vi "EnergyLevelsStatic.vi"(10 "Up/Down Control":bool=TRUE) -> (1 "Energy Level":picture)   [LabVIEW 2023]
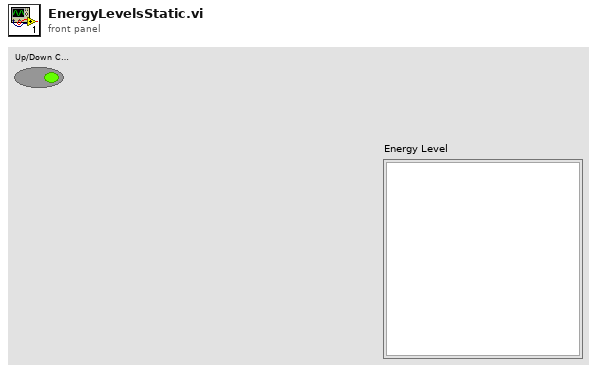
[diagram p1: front panel]
types:
  T1 = cluster{cluster{i32, i32}, cluster{i32, i32}, cluster{i32, i32}, cluster{i32, i32}}
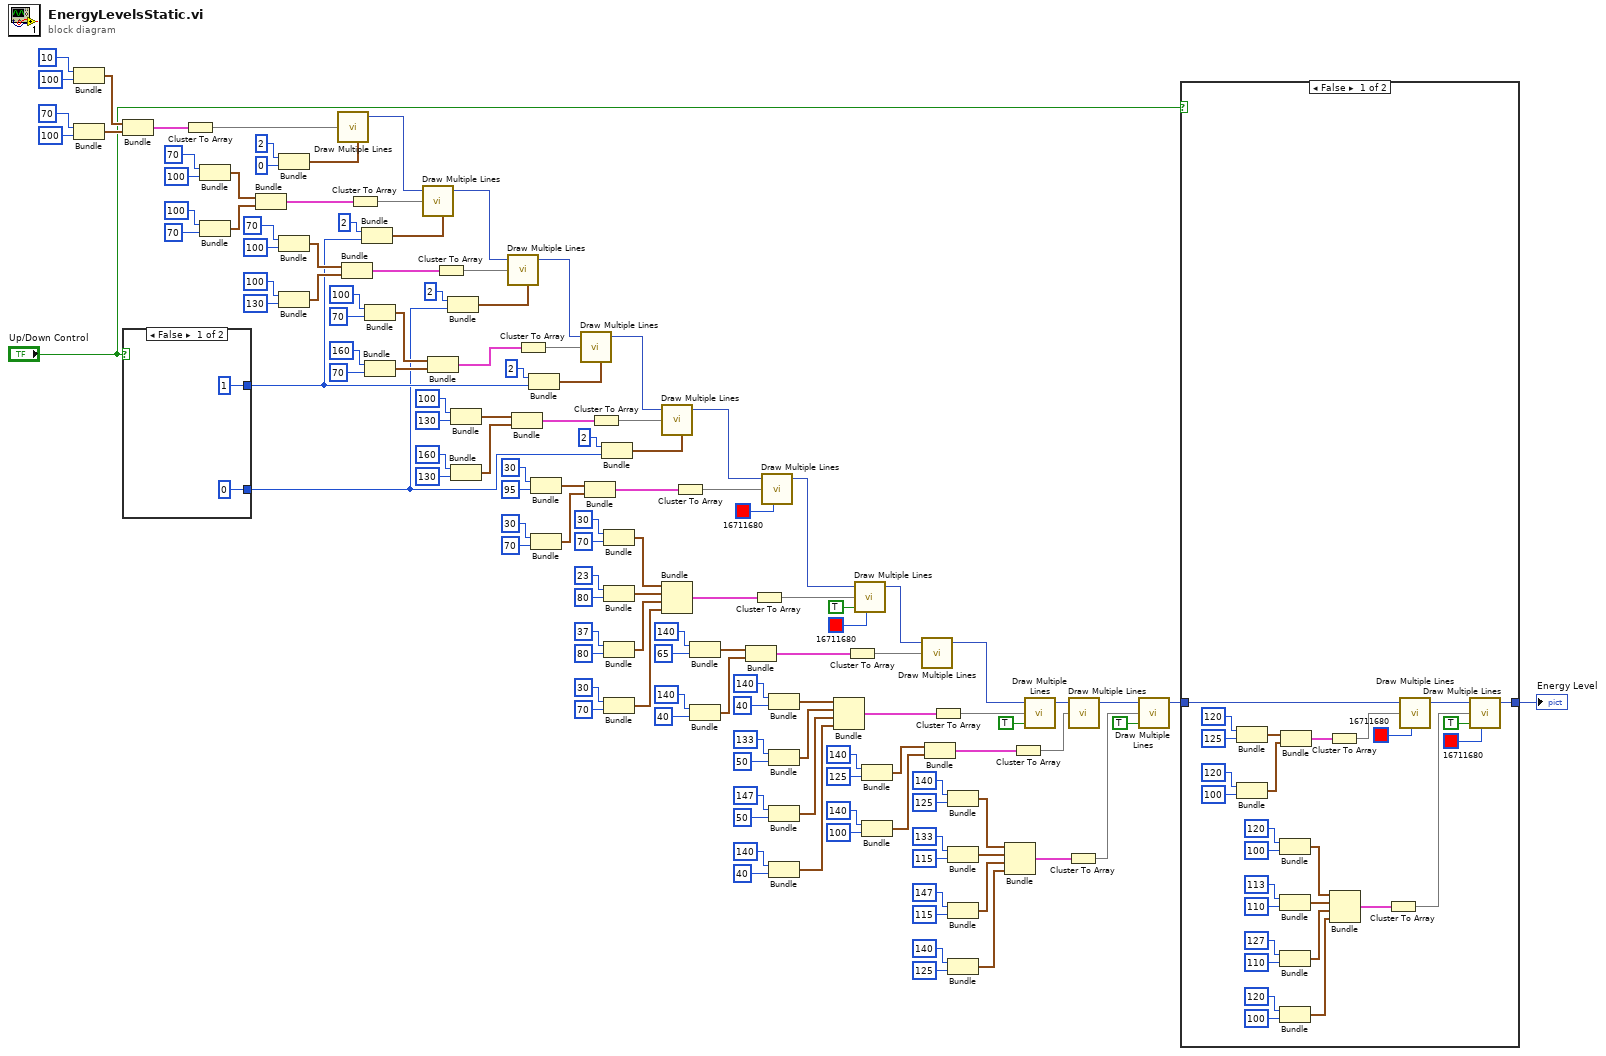
[diagram p0: block diagram]
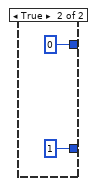
[diagram p2: hidden frame]
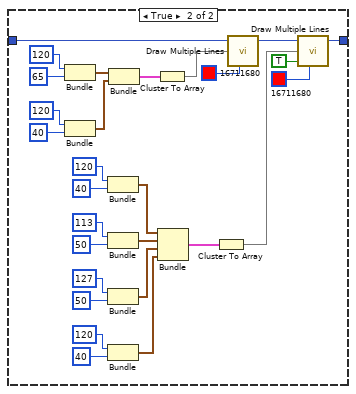
[diagram p3: hidden frame]
diagram:
  n1 = Bundle(10, 100) -> (w137:cluster{i32, i32})  [unwired: 1 in]
  n2 = Bundle(70, 100) -> (w136:cluster{i32, i32})  [unwired: 1 in]
  n3 = Bundle(w137, w136) -> (w130:cluster{cluster{i32, i32}, cluster{i32, i32}})  [unwired: 1 in]
  n4 = case shown="False" "Up/Down Control" {
    tunnel: [1 0] -> w3
    tunnel: [0 1] -> w1
    frame False {
    }
    frame True {
    }
  }
  n5 = Cluster To Array(cluster=w130) -> (array=w131:cluster{i32, i32}[])
  n6 = Bundle(70, 100) -> (w126:cluster{i32, i32})  [unwired: 1 in]
  n7 = Bundle(100, 70) -> (w125:cluster{i32, i32})  [unwired: 1 in]
  n8 = Bundle(w126, w125) -> (w123:cluster{cluster{i32, i32}, cluster{i32, i32}})  [unwired: 1 in]
  n9 = Bundle(2, 0) -> (w129:cluster{i32, i32})  [unwired: 1 in]
  n10 = Bundle(70, 100) -> (w115:cluster{i32, i32})  [unwired: 1 in]
  n11 = Bundle(100, 130) -> (w114:cluster{i32, i32})  [unwired: 1 in]
  n12 = call <vilib>:"Draw Multiple Lines.vi"("line endpoints"=w131, "pen"=w129) -> ("new picture"=w121:picture)  [unwired: 7 in]
  n13 = Bundle(w115, w114) -> (w112:cluster{cluster{i32, i32}, cluster{i32, i32}})  [unwired: 1 in]
  n14 = Cluster To Array(cluster=w123) -> (array=w124:cluster{i32, i32}[])
  n15 = Bundle(2, w3) -> (w120:cluster{i32, i32})  [unwired: 1 in]
  n16 = Bundle(100, 70) -> (w104:cluster{i32, i32})  [unwired: 1 in]
  n17 = Bundle(160, 70) -> (w103:cluster{i32, i32})  [unwired: 1 in]
  n18 = call <vilib>:"Draw Multiple Lines.vi"("picture"=w121, "line endpoints"=w124, "pen"=w120) -> ("new picture"=w105:picture)  [unwired: 6 in]
  n19 = Bundle(w104, w103) -> (w101:cluster{cluster{i32, i32}, cluster{i32, i32}})  [unwired: 1 in]
  n20 = Cluster To Array(cluster=w112) -> (array=w113:cluster{i32, i32}[])
  n21 = Bundle(2, w1) -> (w110:cluster{i32, i32})  [unwired: 1 in]
  n22 = Bundle(100, 130) -> (w93:cluster{i32, i32})  [unwired: 1 in]
  n23 = Bundle(160, 130) -> (w92:cluster{i32, i32})  [unwired: 1 in]
  n24 = call <vilib>:"Draw Multiple Lines.vi"("picture"=w105, "line endpoints"=w113, "pen"=w110) -> ("new picture"=w94:picture)  [unwired: 6 in]
  n25 = Bundle(w93, w92) -> (w90:cluster{cluster{i32, i32}, cluster{i32, i32}})  [unwired: 1 in]
  n26 = Cluster To Array(cluster=w101) -> (array=w102:cluster{i32, i32}[])
  n27 = Bundle(2, w3) -> (w99:cluster{i32, i32})  [unwired: 1 in]
  n28 = Bundle(30, 95) -> (w63:cluster{i32, i32})  [unwired: 1 in]
  n29 = Bundle(30, 70) -> (w62:cluster{i32, i32})  [unwired: 1 in]
  n30 = call <vilib>:"Draw Multiple Lines.vi"("picture"=w94, "line endpoints"=w102, "pen"=w99) -> ("new picture"=w83:picture)  [unwired: 6 in]
  n31 = Bundle(w63, w62) -> (w61:cluster{cluster{i32, i32}, cluster{i32, i32}})  [unwired: 1 in]
  n32 = Cluster To Array(cluster=w90) -> (array=w91:cluster{i32, i32}[])
  n33 = Bundle(2, w1) -> (w88:cluster{i32, i32})  [unwired: 1 in]
  n34 = Bundle(30, 70) -> (w82:cluster{i32, i32})  [unwired: 1 in]
  n35 = Bundle(23, 80) -> (w76:cluster{i32, i32})  [unwired: 1 in]
  n36 = Bundle(37, 80) -> (w73:cluster{i32, i32})  [unwired: 1 in]
  n37 = Bundle(30, 70) -> (w68:cluster{i32, i32})  [unwired: 1 in]
  n38 = call <vilib>:"Draw Multiple Lines.vi"("picture"=w83, "line endpoints"=w91, "pen"=w88) -> ("new picture"=w59:picture)  [unwired: 6 in]
  n39 = Bundle(w82, w76, w73, w68) -> (w66:T1)  [unwired: 1 in]
  n40 = Cluster To Array(cluster=w61) -> (array=w60:cluster{i32, i32}[])
  n41 = Bundle(140, 65) -> (w53:cluster{i32, i32})  [unwired: 1 in]
  n42 = Bundle(140, 40) -> (w54:cluster{i32, i32})  [unwired: 1 in]
  n43 = Bundle(w53, w54) -> (w55:cluster{cluster{i32, i32}, cluster{i32, i32}})  [unwired: 1 in]
  n44 = Cluster To Array(cluster=w66) -> (array=w81:cluster{i32, i32}[])
  n45 = call <vilib>:"Draw Multiple Lines.vi"("picture"=w59, "line endpoints"=w60, "color(black)"=u32 16711680) -> ("new picture"=w58:picture)  [unwired: 6 in]
  n46 = Bundle(140, 40) -> (w48:cluster{i32, i32})  [unwired: 1 in]
  n47 = Bundle(133, 50) -> (w44:cluster{i32, i32})  [unwired: 1 in]
  n48 = Bundle(147, 50) -> (w41:cluster{i32, i32})  [unwired: 1 in]
  n49 = Bundle(140, 40) -> (w36:cluster{i32, i32})  [unwired: 1 in]
  n50 = Bundle(w48, w44, w41, w36) -> (w34:T1)  [unwired: 1 in]
  n51 = Cluster To Array(cluster=w55) -> (array=w56:cluster{i32, i32}[])
  n52 = call <vilib>:"Draw Multiple Lines.vi"("picture"=w58, "line endpoints"=w81, "fill?(F)"=TRUE, "color(black)"=u32 16711680) -> ("new picture"=w57:picture)  [unwired: 5 in]
  n53 = Bundle(140, 125) -> (w14:cluster{i32, i32})  [unwired: 1 in]
  n54 = Bundle(140, 100) -> (w15:cluster{i32, i32})  [unwired: 1 in]
  n55 = call <vilib>:"Draw Multiple Lines.vi"("picture"=w57, "line endpoints"=w56) -> ("new picture"=w33:picture)  [unwired: 7 in]
  n56 = Bundle(w14, w15) -> (w16:cluster{cluster{i32, i32}, cluster{i32, i32}})  [unwired: 1 in]
  n57 = Cluster To Array(cluster=w34) -> (array=w47:cluster{i32, i32}[])
  n58 = Bundle(140, 125) -> (w32:cluster{i32, i32})  [unwired: 1 in]
  n59 = Bundle(133, 115) -> (w28:cluster{i32, i32})  [unwired: 1 in]
  n60 = Bundle(147, 115) -> (w25:cluster{i32, i32})  [unwired: 1 in]
  n61 = Bundle(140, 125) -> (w20:cluster{i32, i32})  [unwired: 1 in]
  n62 = Bundle(w32, w28, w25, w20) -> (w18:T1)  [unwired: 1 in]
  n63 = Cluster To Array(cluster=w16) -> (array=w17:cluster{i32, i32}[])
  n64 = call <vilib>:"Draw Multiple Lines.vi"("picture"=w33, "line endpoints"=w47, "fill?(F)"=TRUE) -> ("new picture"=w9:picture)  [unwired: 6 in]
  n65 = Cluster To Array(cluster=w18) -> (array=w31:cluster{i32, i32}[])
  n66 = call <vilib>:"Draw Multiple Lines.vi"("picture"=w9, "line endpoints"=w17) -> ("new picture"=w8:picture)  [unwired: 7 in]
  n67 = call <vilib>:"Draw Multiple Lines.vi"("picture"=w8, "line endpoints"=w31, "fill?(F)"=TRUE) -> ("new picture"=w7:picture)  [unwired: 6 in]
  n68 = case shown="False" "Up/Down Control" {
    tunnel: w7 -> [w143 w171]
    tunnel: [w142 w170] -> w6
    frame False {
      n69 = Bundle(120, 125) -> (w162:cluster{i32, i32})  [unwired: 1 in]
      n70 = Bundle(120, 100) -> (w161:cluster{i32, i32})  [unwired: 1 in]
      n71 = Bundle(120, 100) -> (w163:cluster{i32, i32})  [unwired: 1 in]
      n72 = Bundle(113, 110) -> (w164:cluster{i32, i32})  [unwired: 1 in]
      n73 = Bundle(127, 110) -> (w165:cluster{i32, i32})  [unwired: 1 in]
      n74 = Bundle(120, 100) -> (w166:cluster{i32, i32})  [unwired: 1 in]
      n75 = Bundle(w162, w161) -> (w160:cluster{cluster{i32, i32}, cluster{i32, i32}})  [unwired: 1 in]
      n76 = Cluster To Array(cluster=w160) -> (array=w159:cluster{i32, i32}[])
      n77 = Bundle(w163, w164, w165, w166) -> (w167:T1)  [unwired: 1 in]
      n78 = Cluster To Array(cluster=w167) -> (array=w168:cluster{i32, i32}[])
      n79 = call <vilib>:"Draw Multiple Lines.vi"("picture"=w143, "line endpoints"=w159, "color(black)"=u32 16711680) -> ("new picture"=w169:picture)  [unwired: 6 in]
      n80 = call <vilib>:"Draw Multiple Lines.vi"("picture"=w169, "line endpoints"=w168, "fill?(F)"=TRUE, "color(black)"=u32 16711680) -> ("new picture"=w142:picture)  [unwired: 5 in]
    }
    frame True {
      n81 = Bundle(120, 65) -> (w194:cluster{i32, i32})  [unwired: 1 in]
      n82 = Bundle(120, 40) -> (w195:cluster{i32, i32})  [unwired: 1 in]
      n83 = Bundle(120, 40) -> (w188:cluster{i32, i32})  [unwired: 1 in]
      n84 = Bundle(113, 50) -> (w185:cluster{i32, i32})  [unwired: 1 in]
      n85 = Bundle(127, 50) -> (w182:cluster{i32, i32})  [unwired: 1 in]
      n86 = Bundle(120, 40) -> (w177:cluster{i32, i32})  [unwired: 1 in]
      n87 = Bundle(w194, w195) -> (w196:cluster{cluster{i32, i32}, cluster{i32, i32}})  [unwired: 1 in]
      n88 = Cluster To Array(cluster=w196) -> (array=w197:cluster{i32, i32}[])
      n89 = Bundle(w188, w185, w182, w177) -> (w176:T1)  [unwired: 1 in]
      n90 = Cluster To Array(cluster=w176) -> (array=w174:cluster{i32, i32}[])
      n91 = call <vilib>:"Draw Multiple Lines.vi"("picture"=w171, "line endpoints"=w197, "color(black)"=u32 16711680) -> ("new picture"=w172:picture)  [unwired: 6 in]
      n92 = call <vilib>:"Draw Multiple Lines.vi"("picture"=w172, "line endpoints"=w174, "fill?(F)"=TRUE, "color(black)"=u32 16711680) -> ("new picture"=w170:picture)  [unwired: 5 in]
    }
  }
  "Energy Level" <- w6
